vi "Table_ScrollaBar.vi"(3 "error in":errorcluster, 4 "Line to focus":string, 5 "TableIn":refnum<vi>) -> (0 "error out":errorcluster, 2 "Tableout":refnum<vi>)   [LabVIEW 2017]
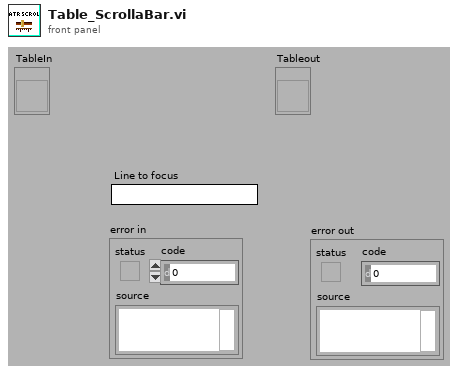
[diagram p1: front panel]
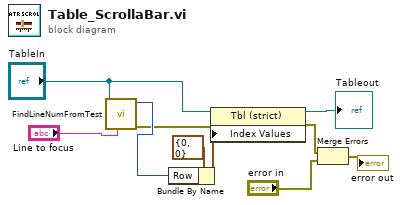
[diagram p0: block diagram]
diagram:
  n1 = call "FindLineNumFromTest.vi"("Test Paragraph"="Line to focus", "TableIn"="TableIn") -> ("error out"=w4:errorcluster, "Line number"=w5:i32)  [unwired: 3 in, 2 out]
  n2 = Bundle By Name(cluster=cluster{"Row":i32, "Column":i32} {"Row"=0, "Column"=0} ("Edit Position"), "Row"=w5) -> (w9:cluster{"Row":i32, "Column":i32})
  n3 = property on="Property Node" class="Tbl (strict)"(reference="TableIn", error in=w4, "Index Values"=w9) -> (reference out=→"Tableout":refnum<vi>, error out=w7:errorcluster)
  n4 = Merge Errors(w7, "error in") -> (→"error out":errorcluster)
